vi "Pre-Process.vi"(11 "Arilou in":refnum<class "Arilou.lvclass">) -> (3 "Arilou out":refnum<class "Arilou.lvclass">)   [LabVIEW 2021, in "Arilou.lvclass"]
uses:
  Arilou.lvclass
  Vector 2D/Vector 2D.lvclass
  Element/Element.lvclass
  Control State/Control State.lvclass
  Ship/Ship.lvclass
  Motion/Motion.lvclass
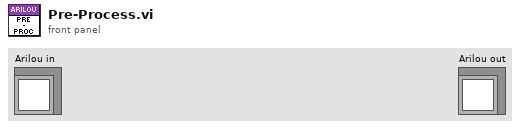
[diagram p1: front panel]
types:
  T1 = typedef "Control State.lvclass/Button State.ctl" = enum16{"Undefined", "Pressed", "Released", "Held", "Not Held"}
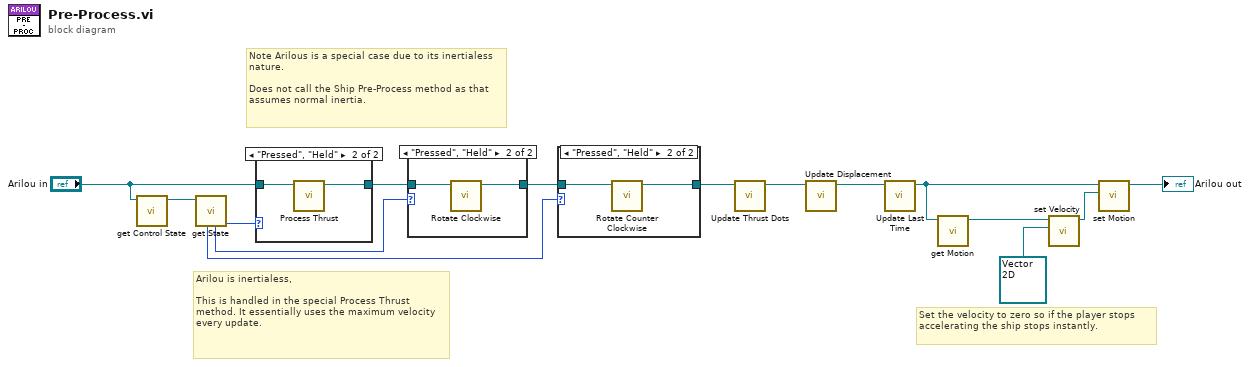
[diagram p0: block diagram]
diagram:
  # "Set the velocity to zero so if the player stops accelerating the ship stops instantly."
  # "Note Arilous is a special case due to its inertialess nature.\n\nDoes not call the Ship Pre-Process method as that assumes normal inertia."
  # "Arilou is inertialess, \n\nThis is handled in the special Process Thrust method. It essentially uses the maximum velocity every update."
  n1 = call "get Control State.vi"("Ship in"="Arilou in") -> ("Control State"=w6:refnum<class "Control State.lvclass">)  [unwired: 10 in]
  n2 = call "get State.vi"("Control State in"=w6) -> ("Thrust"=w13:T1, "Rotate Clockwise"=w12:T1, "Rotate Counter Clockwise"=w9:T1)  [unwired: 6 in, 2 out]
  n3 = case shown="\"Pressed\", \"Held\"" w13 {
    tunnel: "Arilou in" -> [w16 w17]
    tunnel: [w16 w18] -> w11
    frame Default {
    }
    frame "Pressed", "Held" {
      n4 = call "Process Thrust.vi"("Arilou in"=w17) -> ("Arilou out"=w18:refnum<class "Arilou.lvclass">)  [unwired: 10 in]
    }
  }
  n5 = case shown="\"Pressed\", \"Held\"" w12 {
    tunnel: w11 -> [w19 w21]
    tunnel: [w19 w20] -> w10
    frame Default {
    }
    frame "Pressed", "Held" {
      n6 = call "Rotate Clockwise.vi"("Element in"=w21) -> ("Element out"=w20:refnum<class "Arilou.lvclass">)  [unwired: 10 in]
    }
  }
  n7 = case shown="\"Pressed\", \"Held\"" w9 {
    tunnel: w10 -> [w22 w24]
    tunnel: [w22 w23] -> w14
    frame Default {
    }
    frame "Pressed", "Held" {
      n8 = call "Rotate Counter Clockwise.vi"("Element in"=w24) -> ("Element out"=w23:refnum<class "Arilou.lvclass">)  [unwired: 10 in]
    }
  }
  n9 = call "Update Thrust Dots.vi"("Ship in"=w14) -> ("Ship out"=w8:refnum<class "Arilou.lvclass">)  [unwired: 10 in]
  n10 = call "Update Displacement.vi"("Element in"=w8) -> ("Element out"=w15:refnum<class "Arilou.lvclass">)  [unwired: 10 in]
  n11 = call "Update Last Time.vi"("Element in"=w15) -> ("Element out"=w4:refnum<class "Arilou.lvclass">)  [unwired: 10 in]
  n12 = call "get Motion.vi"("Element in"=w4) -> ("Motion"=w5:refnum<class "Motion.lvclass">)  [unwired: 10 in]
  n13 = call "set Velocity.vi"("Velocity"=refnum<class "Vector 2D.lvclass"> refnum, "Motion in"=w5) -> ("Motion out"=w2:refnum<class "Motion.lvclass">)  [unwired: 9 in]
  n14 = call "set Motion.vi"("Motion"=w2, "Element in"=w4) -> ("Element out"=→"Arilou out":refnum<class "Arilou.lvclass">)  [unwired: 9 in]
